vi "Create Bad Regex.vi"(8 "error in (no error)":errorcluster, 10 "Bad Value":T1) -> (0 "error out":errorcluster, 3 "Bad Regex out":refnum<class "Bad Regex.lvclass">)   [LabVIEW 2020, in "ase.test.lvlib" / "Bad Regex.lvclass"]
uses:
  Bad Regex.lvclass
  Bad Value.ctl
  Bad Regex.lvclass/Bad Regex.ctl
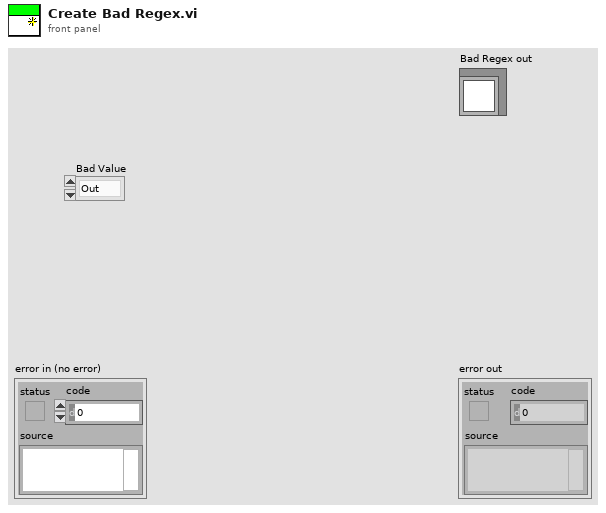
[diagram p1: front panel]
types:
  T1 = typedef "ase.test.lvlib/Bad Regex.lvclass/Bad Value.ctl" = enum16{"Out", "Err", "Both"}
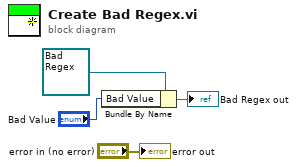
[diagram p0: block diagram]
diagram:
  n1 = Bundle By Name(cluster=refnum<class "Bad Regex.lvclass"> refnum ("serenial.io-ase.test.lvlib:Bad Regex.lvclass"), "Bad Value"="Bad Value") -> (→"Bad Regex out":refnum<class "Bad Regex.lvclass">)
  "error out" <- "error in (no error)"
